vi "太阳能控制器MPPT24.vi"() -> ()   [LabVIEW 2016, in "环境动力监测库.lvlib"]
uses:
  <vilib>/Utility/miscctls.llb/LVPointTypeDef.ctl
  <vilib>/Utility/config.llb/NI_LVConfig.lvlib
  <vilib>/ptbypt/NI_PtbyPt.lvlib
panel:
  out "串口":string
  in  "串口启用 2":bool caption="串口启用"
  in  "报警设置":bool
  in  "MPPT-24 串口":refnum<visa-resource-name> caption="MPPT-24"
  out "充放电信息 2":T1 caption="充放电信息_KWH" {"总累计充电量" format="%.2f"; "当年累计充电量" format="%.2f"; "当月累计充电量" format="%.2f"; "当日累计充电量" format="%.2f"; "当年累计用电量" format="%.2f"; "当月累计用电量" format="%.2f"; "当日累计用电量" format="%.2f"}
  out "状态 2":string caption="状态"
  out "通讯状态 3":bool
  out "控制器信息 2":cluster{"设备温度℃":dbl} caption="控制器信息"
  out "直流负载信息 2":cluster{"负载电压V":dbl, "负载电流A":dbl, "负载功率W":dbl} caption="直流负载信息"
  out "蓄电池信息 2":T2 caption="蓄电池信息"
  out "阵列信息 2":cluster{"阵列电压V":dbl, "阵列电流A":dbl, "发电功率W":dbl} caption="阵列信息"
  # "MPPT-24"
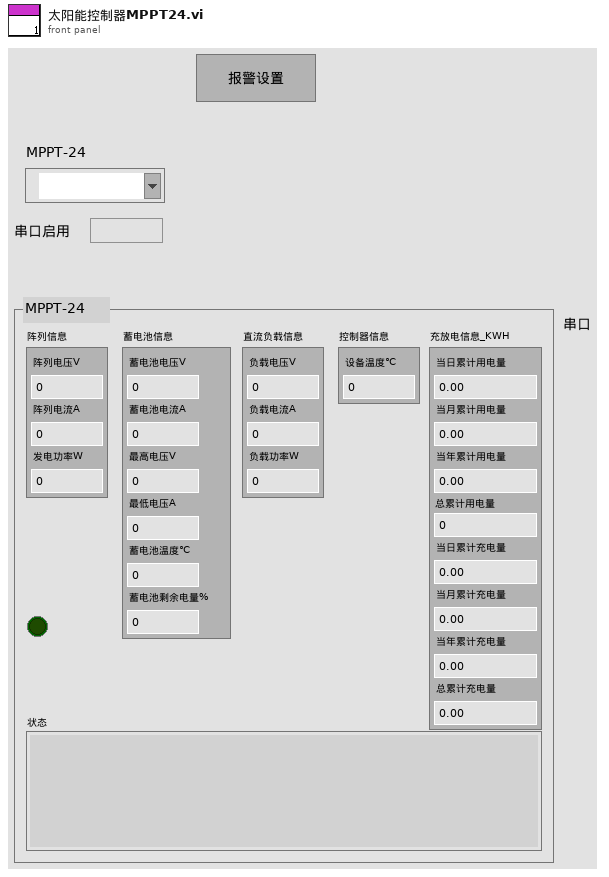
[diagram p1: front panel]
types:
  T1 = cluster{"当日累计用电量":sgl, "当月累计用电量":sgl, "当年累计用电量":sgl, "总累计用电量":sgl, "当日累计充电量":sgl, "当月累计充电量":sgl, "当年累计充电量":sgl, "总累计充电量":sgl}
  T2 = cluster{"蓄电池电压V":dbl, "蓄电池电流A":dbl, "最高电压V":dbl, "最低电压A":dbl, "蓄电池温度℃":dbl, "蓄电池剩余电量%":dbl}
  T3 = cluster{"baud rate (bps)":u32, "stop bits":u16, "parity":u16, "flow control":u16, "timeout":u32, "retries":i32}
  T4 = cluster{"监测项描述:输出":string, "连接方式":enum16{"串口", "TCP"}, "端口":string, "IP address:":string, "Port:":string, "站号":u64, "传感器型号":string, "波特率":u64, "data bits":u64, "停止位":u16, "奇偶校验":u16}
  T5 = typedef "LVPointTypeDef.ctl" = cluster{"Horizontal":i16, "Vertical":i16}
  T6 = cluster{"漏水监测输出":cluster{"漏水监测告警":bool, "告警内容":string}, "门禁监测输出":cluster{"门禁监测告警":bool, "告警内容":string}, "门禁监测输出2":cluster{"门禁监测告警":bool, "告警内容":string}, "温湿度监测输出":cluster{"温湿度监测告警":bool, "告警内容":string}, "烟雾监测输出":cluster{"烟雾监测告警":bool, "告警内容":string}, "空调监测输出":cluster{"空调监测告警":bool, "告警内容":string}, "自动重合闸输出":cluster{"自动重合闸告警":bool, "告警内容":string}, "红外入侵输出":cluster{"红外入侵告警":bool, "告警内容":string}, "振动输出":cluster{"振动告警":bool, "告警内容":string}, "UPS输出":cluster{"UPS告警":bool, "告警内容":string}, "蓄电池输出":cluster{"蓄电池告警":bool, "告警内容":string}, "蓄电池输出2":cluster{"蓄电池告警":bool, "告警内容":string}, "GPS输出":cluster{"定位告警":bool, "告警内容":string}, "北斗输出":cluster{"定位告警":bool, "告警内容":string}, "气象输出":cluster{"气象告警":bool, "告警内容":string}}
  T7 = cluster{"时间":timestamp, "阵列电压_V":dbl, "阵列电流_A":dbl, "发电功率_W":dbl, "蓄电池电压_V":dbl, "蓄电池电流_A":dbl, "最高电压_V":dbl, "最低电压_A":dbl, "蓄电池温度_℃":dbl, "蓄电池剩余电量_%":dbl, "负载电压_V":dbl, "负载电流_A":dbl, "负载功率_W":dbl, "设备温度_℃":dbl, "当日累计用电量_KWH":dbl, "当月累计用电量_KWH":dbl, "当年累计用电量_KWH":dbl, "总累计用电量_KWH":dbl, "当日累计充电量_KWH":dbl, "当月累计充电量_KWH":dbl, "当年累计充电量_KWH":dbl, "总累计充电量_KWH":dbl}
  T8 = typedef "LVDateTimeRec.ctl" = cluster{"秒数的小数部分":dbl, "秒":i32, "分":i32, "时":i32, "日":i32, "月":i32, "年":i32, "天数（周）":i32, "天数（年）":i32, "DST":i32}
  T9 = cluster{"市电":cluster{"状态":bool, "电压:":u16, "电流：":dbl, "详情  ":bool}, "UPS":cluster{"状态":bool, "输入电压:":sgl, "输出电压:":sgl, "电池电量:":u8, "电量":u16, "详情  ":bool}, "蓄电池12V":cluster{"状态":bool, "电压:":sgl, "电流:":sgl, "电池电量:":u8, "电量":u16, "详情  ":bool}, "蓄电池24V":cluster{"状态":bool, "电压:":sgl, "电流:":sgl, "电池电量:":u8, "电量":u16, "详情  ":bool}}
  T10 = cluster{"状态":cluster{"蓄电池状态":string, "阵列状态":string, "充电状态":string, "负载状态":string, "设备状态":string}, "充放电信息":cluster{"当日累计用电量":sgl, "当月累计用电量":sgl, "当年累计用电量":sgl, "总累计用电量":sgl, "当日累计充电量":sgl, "当月累计充电量":sgl, "当年累计充电量":sgl, "总累计充电量":sgl}, "控制器信息":cluster{"设备温度℃":dbl}, "蓄电池信息":cluster{"蓄电池电压V":dbl, "蓄电池电流A":dbl, "最高电压V":dbl, "最低电压A":dbl, "蓄电池温度℃":dbl, "蓄电池剩余电量%":dbl}, "阵列信息":cluster{"阵列电压V":dbl, "阵列电流A":dbl, "发电功率W":dbl}, "直流负载信息":cluster{"负载电压V":dbl, "负载电流A":dbl, "负载功率W":dbl}, "error out":errorcluster}
  T11 = enum32{"Bad", "Idle", "Run top level", "Running"}
  T12 = typedef "NI_LVConfig.lvlib/Config Data RefNum.ctl" = refnum<k1>
  T13 = enum8{"Enabled", "Disabled", "Disabled and Grayed Out"}
  T14 = cluster{"蓄电池状态":string, "阵列状态":string, "充电状态":string, "负载状态":string, "设备状态":string}
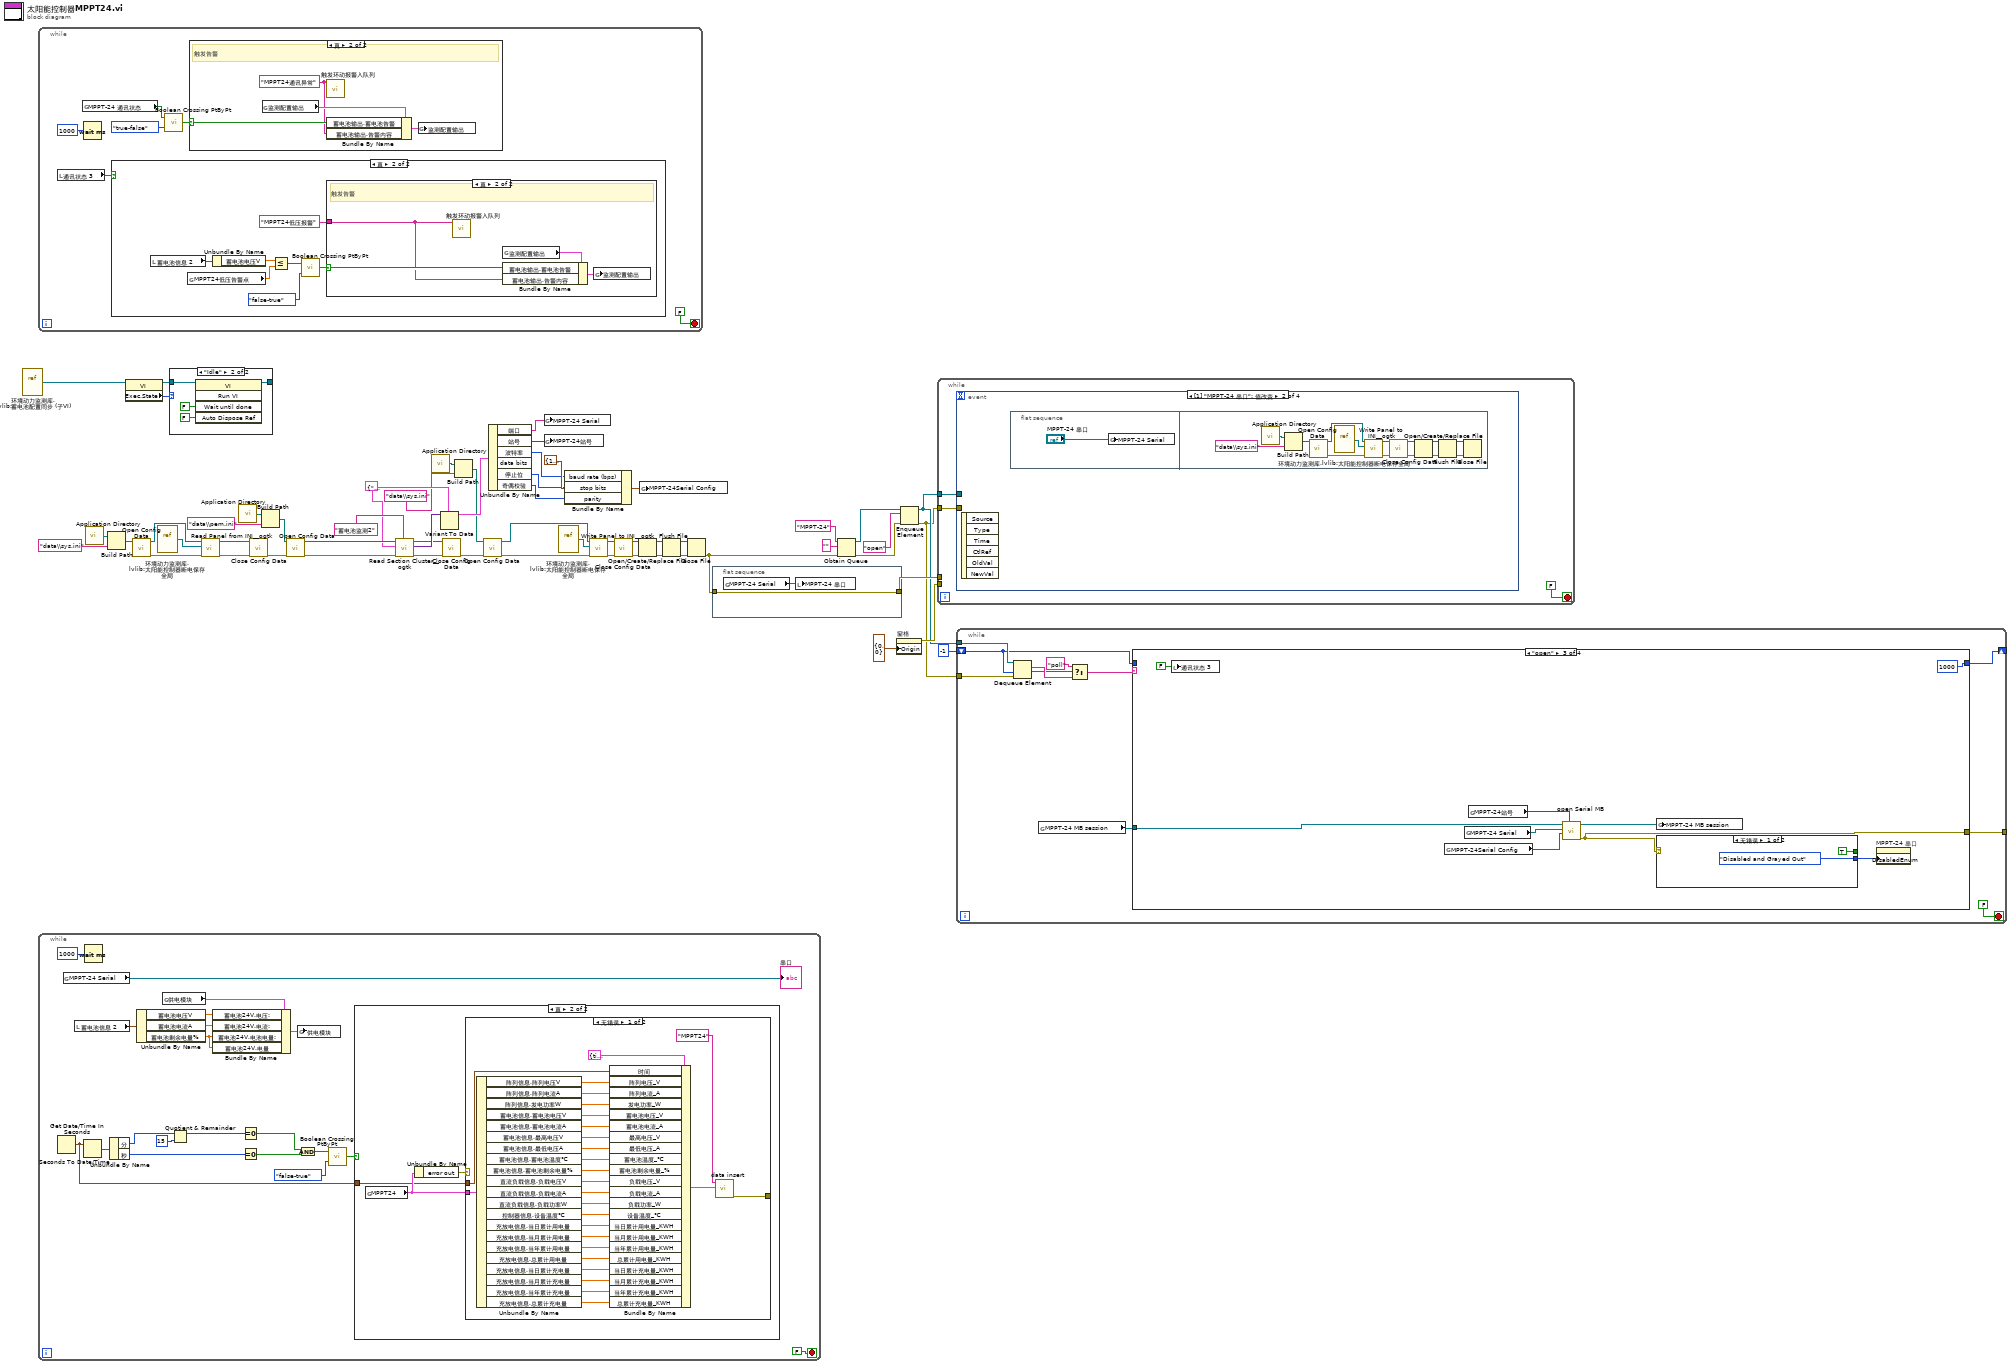
[diagram p0: block diagram]
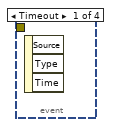
[diagram p8: hidden frame]
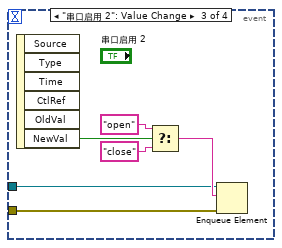
[diagram p9: hidden frame]
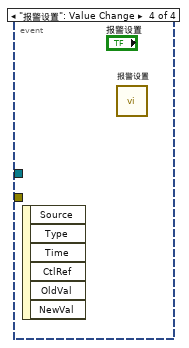
[diagram p10: hidden frame]
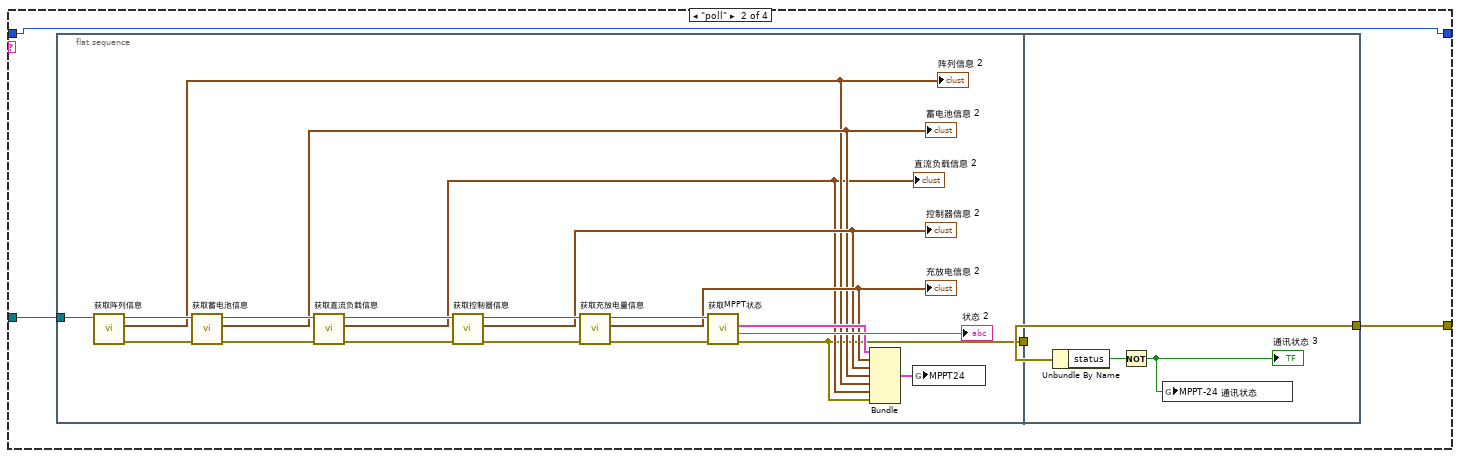
[diagram p12: hidden frame]
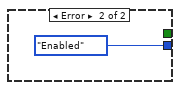
[diagram p13: hidden frame]
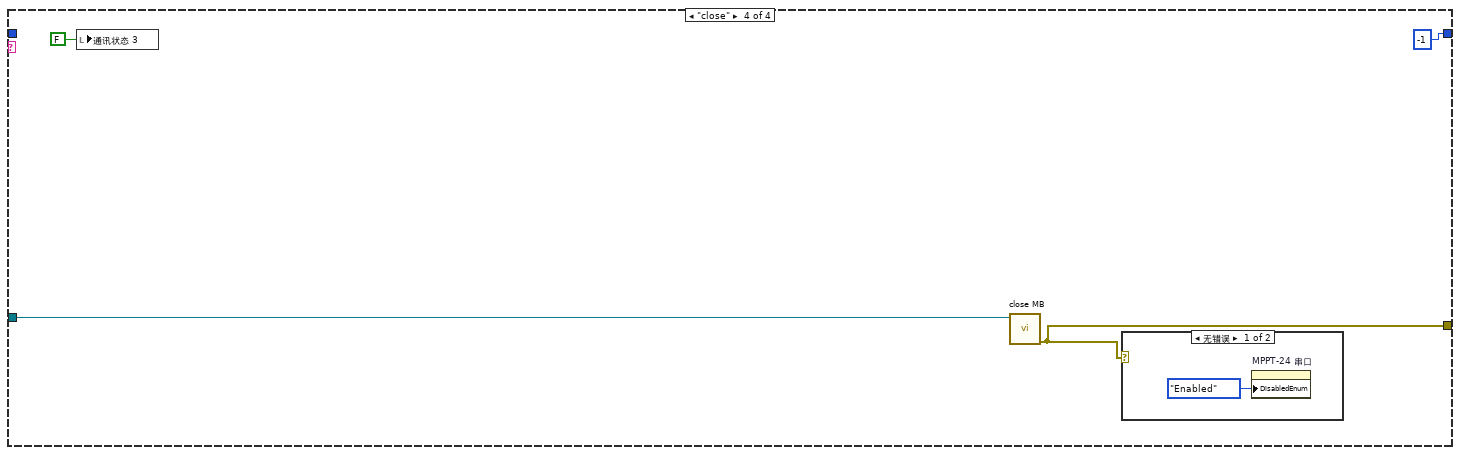
[diagram p14: hidden frame]
diagram:
  w36 = T4 {"监测项描述:输出"="", "连接方式"=enum."串口", "端口"="", "IP address:"="", "Port:"="", "站号"=19200, "传感器型号"="", "波特率"=19200, "data bits"=8, "停止位"=10, "奇偶校验"=0} ("输入簇")
  n1 = vi-ref "环境动力监测库.lvlib:蓄电池配置同步 (子VI).vi"() -> (w7:refnum<vi>)
  n2 = while {
    stop <- FALSE stop-if-true
    n3 = local read "通讯状态 3"() -> (w61:bool)
    n4 = global read "太阳能控制器全局.vi" "MPPT-24 通讯状态"() -> (w58:bool)
    n5 = Wait (ms)(milliseconds to wait=u32 1000 ("等待时间（毫秒）")) -> ()  [unwired: 1 out]
    n6 = case shown="真" w61 {
      frame False {
      }
      frame True {
        n7 = local read "蓄电池信息 2"() -> (w74:T2)
        n8 = global read "太阳能控制器断电保存全局.vi" "MPPT24低压告警点"() -> (w70:dbl)
        n9 = Unbundle By Name(w74) -> ("蓄电池电压V"=w71:dbl)
        n10 = Less Or Equal?(x=w71, y=w70) -> (x <= y?=w69:bool)
        n11 = call <vilib>:"Boolean Crossing PtByPt.vi"("direction"=enum16{"either", "false-true", "true-false"}."false-true", "input"=w69) -> ("crossing"=w72:bool)  [unwired: 1 in]
        n12 = case shown="真" w72 {
          selector: w72 -> [_ w76]
          tunnel: "MPPT24低压报警" ("设备") -> [_ w75]
          frame False {
          }
          frame True {
            # "触发告警"
            n13 = call "触发环动报警入队列.vi"("报警内容"=w75) -> ()  [unwired: 11 in]
            n14 = global read "断电保存全局变量.vi" "监测配置输出"() -> (w77:T6)
            n15 = Bundle By Name(cluster=w77, "蓄电池输出.蓄电池告警"=w76, "蓄电池输出.告警内容"=w75) -> (w78:T6)
            n16 = global write "断电保存全局变量.vi" "监测配置输出"(w78) -> ()
          }
        }
      }
    }
    n17 = call <vilib>:"Boolean Crossing PtByPt.vi"("direction"=enum16{"either", "false-true", "true-false"}."true-false", "input"=w58) -> ("crossing"=w59:bool)  [unwired: 1 in]
    n18 = case shown="真" w59 {
      selector: w59 -> [_ w65]
      frame False {
      }
      frame True {
        w64 = "MPPT24通讯异常" ("报警内容")
        # "触发告警"
        n19 = global read "断电保存全局变量.vi" "监测配置输出"() -> (w67:T6)
        n20 = call "触发环动报警入队列.vi"("报警内容"=w64) -> ()  [unwired: 11 in]
        n21 = Bundle By Name(cluster=w67, "蓄电池输出.蓄电池告警"=w65, "蓄电池输出.告警内容"=w64) -> (w66:T6)
        n22 = global write "断电保存全局变量.vi" "监测配置输出"(w66) -> ()
      }
    }
  }
  n23 = while {
    stop <- FALSE stop-if-true
    n24 = Get Date/Time In Seconds() -> (seconds since 1Jan1904=w86:timestamp)
    n25 = global read "太阳能控制器断电保存全局.vi" "MPPT-24 Serial"() -> (→"串口":refnum<visa-resource-name>)
    n26 = local read "蓄电池信息 2"() -> (w82:T2)
    n27 = Seconds To Date/Time(time stamp (now)=w86) -> (date time rec=w96:T8)  [unwired: 1 in]
    n28 = Wait (ms)(milliseconds to wait=u32 1000 ("等待时间（毫秒）")) -> ()  [unwired: 1 out]
    n29 = Unbundle By Name(w96) -> ("分"=w95:i32, "秒"=w92:i32)
    n30 = Unbundle By Name(w82) -> ("蓄电池电压V"=w81:dbl, "蓄电池电流A"=w80:dbl, "蓄电池剩余电量%"=w79:dbl)
    n31 = global read "内部交互全局变量.vi" "供电模块"() -> (w84:T9)
    n32 = Quotient & Remainder(x=w95, y=15) -> (x-y*floor(x/y)=w93:i32)  [unwired: 1 out]
    n33 = Bundle By Name(cluster=w84, "蓄电池24V.电压:"=w81, "蓄电池24V.电流:"=w80, "蓄电池24V.电池电量:"=w79, "蓄电池24V.电量"=w79) -> (w83:T9)
    n34 = Equal To 0?(x=w93) -> (x = 0?=w91:bool)
    n35 = Equal To 0?(x=w92) -> (x = 0?=w90:bool)
    n36 = global write "内部交互全局变量.vi" "供电模块"(w83) -> ()
    n37 = And(x=w91, y=w90) -> (x .and. y?=w89:bool)
    n38 = call <vilib>:"Boolean Crossing PtByPt.vi"("direction"=enum16{"either", "false-true", "true-false"}."false-true", "input"=w89) -> ("crossing"=w87:bool)  [unwired: 1 in]
    n39 = case shown="真" w87 {
      tunnel: w86 -> [_ w99]
      frame False {
      }
      frame True {
        n40 = global read "太阳能控制器全局.vi" "MPPT24"() -> (w101:T10)
        n41 = Unbundle By Name(w101) -> ("error out"=w100:errorcluster)
        n42 = case shown="无错误" w100 {
          tunnel: w101 -> [w106 _]
          tunnel: w99 -> [w105 _]
          tunnel: [w102 _] -> _
          frame No Error {
            n43 = Unbundle By Name(w106) -> ("阵列信息.阵列电压V"=w108:dbl, "阵列信息.阵列电流A"=w109:dbl, "阵列信息.发电功率W"=w110:dbl, "蓄电池信息.蓄电池电压V"=w111:dbl, "蓄电池信息.蓄电池电流A"=w112:dbl, "蓄电池信息.最高电压V"=w113:dbl, "蓄电池信息.最低电压A"=w114:dbl, "蓄电池信息.蓄电池温度℃"=w115:dbl, "蓄电池信息.蓄电池剩余电量%"=w116:dbl, "直流负载信息.负载电压V"=w117:dbl, "直流负载信息.负载电流A"=w118:dbl, "直流负载信息.负载功率W"=w119:dbl, "控制器信息.设备温度℃"=w120:dbl, "充放电信息.当日累计用电量"=w121:sgl, "充放电信息.当月累计用电量"=w122:sgl, "充放电信息.当年累计用电量"=w123:sgl, "充放电信息.总累计用电量"=w124:sgl, "充放电信息.当日累计充电量"=w125:sgl, "充放电信息.当月累计充电量"=w126:sgl, "充放电信息.当年累计充电量"=w127:sgl, "充放电信息.总累计充电量"=w128:sgl)
            n44 = Bundle By Name(cluster=T7 {"时间"=timestamp(0 s since 1904-01-01), "阵列电压_V"=0.0, "阵列电流_A"=0.0, "发电功率_W"=0.0, "蓄电池电压_V"=0.0, "蓄电池电流_A"=0.0, "最高电压_V"=0.0, "最低电压_A"=0.0, "蓄电池温度_℃"=0.0, "蓄电池剩余电量_%"=0.0, "负载电压_V"=0.0, "负载电流_A"=0.0, "负载功率_W"=0.0, "设备温度_℃"=0.0, "当日累计用电量_KWH"=0.0, "当月累计用电量_KWH"=0.0, "当年累计用电量_KWH"=0.0, "总累计用电量_KWH"=0.0, "当日累计充电量_KWH"=0.0, "当月累计充电量_KWH"=0.0, "当年累计充电量_KWH"=0.0, "总累计充电量_KWH"=0.0} ("data in"), "时间"=w105, "阵列电压_V"=w108, "阵列电流_A"=w109, "发电功率_W"=w110, "蓄电池电压_V"=w111, "蓄电池电流_A"=w112, "最高电压_V"=w113, "最低电压_A"=w114, "蓄电池温度_℃"=w115, "蓄电池剩余电量_%"=w116, "负载电压_V"=w117, "负载电流_A"=w118, "负载功率_W"=w119, "设备温度_℃"=w120, "当日累计用电量_KWH"=w121, "当月累计用电量_KWH"=w122, "当年累计用电量_KWH"=w123, "总累计用电量_KWH"=w124, "当日累计充电量_KWH"=w125, "当月累计充电量_KWH"=w126, "当年累计充电量_KWH"=w127, "总累计充电量_KWH"=w128) -> (w104:T7)
            n45 = call "data insert.vi"("data in"=w104, "table"="MPPT24") -> ("error out"=w102:errorcluster)  [unwired: 9 in]
          }
          frame Error {
          }
        }
      }
    }
  }
  n46 = call <vilib>:"Application Directory.vi"() -> ("Application Directory"=w13:path)
  n47 = Build Path(base path=w13, name or relative path="data\\sys.ini" ("名称或相对路径")) -> (appended path=w12:path)
  n48 = property class="VI"(reference=w7) -> (reference out=w8:refnum<vi>, "Exec.State"=w9:T11)  [unwired: 1 in, 1 out]
  n49 = call <vilib>:"Open Config Data.vi"("configuration file path"=w12) -> ("error out"=w16:errorcluster, "refnum"=w15:T12)  [unwired: 8 in, 1 out]
  n50 = vi-ref "环境动力监测库.lvlib:太阳能控制器断电保存全局.vi"() -> (w11:refnum<vi>)
  n51 = case shown="\"Idle\"" w9 {
    tunnel: w8 -> [w129 w131]
    tunnel: [w129 w130] -> _
    frame "Bad", Default {
    }
    frame "Idle" {
      n52 = invoke class="VI" method="Run VI"(reference=w131, "Wait until done"=FALSE ("结束前等待"), "Auto Dispose Ref"=FALSE ("自动销毁引用")) -> (reference out=w130:refnum<vi>)  [unwired: 2 in, 4 out]
    }
  }
  n53 = call <userlib>:"Read Panel from INI__ogtk.vi"("error in (no error)"=w16, "VI ref"=w11, "refnum"=w15) -> ("error out"=w18:errorcluster, "refnum out"=w17:T12)  [unwired: 7 in]
  n54 = call <vilib>:"Application Directory.vi"() -> ("Application Directory"=w40:path)
  n55 = call <vilib>:"Close Config Data.vi"("error in (no error)"=w18, "refnum"=w17) -> ("error out"=w10:errorcluster)  [unwired: 8 in, 1 out]
  n56 = Build Path(base path=w40, name or relative path="data\\pem.ini" ("名称或相对路径")) -> (appended path=w39:path)
  n57 = call <vilib>:"Open Config Data.vi"("error in (no error)"=w10, "configuration file path"=w39) -> ("error out"=w38:errorcluster, "refnum"=w37:T12)  [unwired: 7 in, 1 out]
  n58 = call <userlib>:"Read Section Cluster__ogtk.vi"("section (optional)"="蓄电池监测2", "error in (no error)"=w38, "Section Formatted Cluster Type"=w36, "refnum"=w37) -> ("error out"=w44:errorcluster, "Section Formatted Cluster"=w45:variant, "dup refnum"=w43:T12)  [unwired: 3 in, 2 out]
  n59 = call <vilib>:"Application Directory.vi"() -> ("Application Directory"=w34:path)
  n60 = Variant To Data(type=w36, Variant=w45) -> (data=w46:T4)  [unwired: 1 in, 1 out]
  n61 = call <vilib>:"Close Config Data.vi"("error in (no error)"=w44, "refnum"=w43) -> ("error out"=w22:errorcluster)  [unwired: 8 in, 1 out]
  n62 = Build Path(base path=w34, name or relative path="data\\sys.ini" ("名称或相对路径")) -> (appended path=w33:path)
  n63 = call <vilib>:"Open Config Data.vi"("error in (no error)"=w22, "configuration file path"=w33) -> ("error out"=w30:errorcluster, "refnum"=w32:T12)  [unwired: 7 in, 1 out]
  n64 = Unbundle By Name(w46) -> ("端口"=w20:string, "站号"=w5:u64, "波特率"=w4:u64, "停止位"=w3:u16, "奇偶校验"=w2:u16)  [unwired: 1 out]
  n65 = global write "太阳能控制器断电保存全局.vi" "MPPT-24 Serial"(w20) -> ()
  n66 = global write "太阳能控制器断电保存全局.vi" "MPPT-24站号"(w5) -> ()
  n67 = vi-ref "环境动力监测库.lvlib:太阳能控制器断电保存全局.vi"() -> (w21:refnum<vi>)
  n68 = Bundle By Name(cluster=T3 {"baud rate (bps)"=115200, "stop bits"=10, "parity"=0, "flow control"=0, "timeout"=1000, "retries"=1} ("MPPT-24Serial Config"), "baud rate (bps)"=w4, "stop bits"=w3, "parity"=w2) -> (w1:T3)
  n69 = call <userlib>:"Write Panel to INI__ogtk.vi"("error in (no error)"=w30, "VI ref"=w21, "refnum"=w32) -> ("error out"=w29:errorcluster, "refnum out"=w31:T12)  [unwired: 7 in]
  n70 = call <vilib>:"Close Config Data.vi"("error in (no error)"=w29, "refnum"=w31) -> ("error out"=w24:errorcluster, "file path"=w23:path)  [unwired: 8 in]
  n71 = Open/Create/Replace File(file path (use dialog)=w23, error in=w24) -> (refnum out=w27:refnum<file>, error out=w28:errorcluster)  [unwired: 4 in, 1 out]
  n72 = global write "太阳能控制器断电保存全局.vi" "MPPT-24Serial Config"(w1) -> ()
  n73 = Flush File(refnum=w27, error in=w28) -> (refnum out=w26:refnum<file>, error out=w25:errorcluster)
  n74 = Close File(refnum=w26, error in=w25) -> (error out=w19:errorcluster)  [unwired: 1 out]
  n75 = flat-sequence {
    tunnel: w19 -> [w134]
    tunnel: [w134] -> w49
    frame #0 {
      n76 = global read "太阳能控制器断电保存全局.vi" "MPPT-24 Serial"() -> (w135:refnum<visa-resource-name>)
      n77 = local write "MPPT-24 串口"(w135) -> ()
    }
  }
  n78 = Obtain Queue(name (unnamed)="MPPT-24" ("名称（未命名）"), element data type="", error in (no error)=w19) -> (queue out=w51:refnum<queue>, error out=w50:errorcluster)  [unwired: 2 in, 1 out]
  n79 = property on="窗格" class="Pane"("Origin"=T5 {"Horizontal"=0, "Vertical"=0} ("原点")) -> (error out=w55:errorcluster)  [unwired: 2 in, 1 out]
  n80 = Enqueue Element(queue=w51, element="open" ("元素"), error in (no error)=w50) -> (queue out=w48:refnum<queue>, error out=w47:errorcluster)  [unwired: 1 in, 1 out]
  n81 = while {
    tunnel: w55 -> [_]
    tunnel: w49 -> [_]
    tunnel: w48 -> [w137]
    tunnel: w47 -> [w136]
    stop <- FALSE stop-if-true
    n82 = event shown="[1] \"MPPT-24 串口\": 值改变" {
      selector: _ -> [_ _ _ _]
      dyn-events: _ -> [_ _ _ _]
      timeout: _ -> [_ _ _ _]
      tunnel: w137 -> [_ _ w155 _]
      tunnel: w136 -> [_ _ w154 _]
      event Timeout {
        n83 = event-data() -> ()  [unwired: 1 in, 3 out]
      }
      event "MPPT-24 串口": Value Change {
        n84 = event-data() -> ()  [unwired: 1 in, 6 out]
        n85 = flat-sequence {
          frame #0 {
            n86 = global write "太阳能控制器断电保存全局.vi" "MPPT-24 Serial"("MPPT-24 串口") -> ()
          }
          frame #1 {
            n87 = call <vilib>:"Application Directory.vi"() -> ("Application Directory"=w153:path)
            n88 = Build Path(base path=w153, name or relative path="data\\sys.ini" ("名称或相对路径")) -> (appended path=w151:path)
            n89 = call <vilib>:"Open Config Data.vi"("configuration file path"=w151) -> ("error out"=w147:errorcluster, "refnum"=w150:T12)  [unwired: 8 in, 1 out]
            n90 = vi-ref "环境动力监测库.lvlib:太阳能控制器断电保存全局.vi"() -> (w149:refnum<vi>)
            n91 = call <userlib>:"Write Panel to INI__ogtk.vi"("error in (no error)"=w147, "VI ref"=w149, "refnum"=w150) -> ("error out"=w146:errorcluster, "refnum out"=w148:T12)  [unwired: 7 in]
            n92 = call <vilib>:"Close Config Data.vi"("error in (no error)"=w146, "refnum"=w148) -> ("error out"=w141:errorcluster, "file path"=w140:path)  [unwired: 8 in]
            n93 = Open/Create/Replace File(file path (use dialog)=w140, error in=w141) -> (refnum out=w144:refnum<file>, error out=w145:errorcluster)  [unwired: 4 in, 1 out]
            n94 = Flush File(refnum=w144, error in=w145) -> (refnum out=w143:refnum<file>, error out=w142:errorcluster)
            n95 = Close File(refnum=w143, error in=w142) -> ()  [unwired: 2 out]
          }
        }
      }
      event "串口启用 2": Value Change {
        n96 = event-data() -> ("NewVal"=w156:bool)  [unwired: 1 in, 5 out]
        n97 = Select(t="open", s=w156, f="close") -> (s? t:f=w158:string)
        n98 = Enqueue Element(queue=w155, element=w158, error in (no error)=w154) -> ()  [unwired: 1 in, 3 out]
      }
      event "报警设置": Value Change {
        n99 = event-data() -> ()  [unwired: 1 in, 6 out]
        n100 = call "报警设置.vi"() -> ()  [unwired: 12 in]
      }
    }
  }
  n101 = while {
    tunnel: w48 -> [w167]
    tunnel: w47 -> [w166]
    shift-right: [w162] -> _
    shift-left: -1 ("超时毫秒(-1)") -> [w160]
    tunnel: [w163] -> _
    stop <- FALSE stop-if-true
    n102 = Dequeue Element(queue=w167, timeout in ms (-1)=w160, error in (no error)=w166) -> (element=w170:string, timed out?=w168:bool)  [unwired: 2 out]
    n103 = global read "太阳能控制器全局.vi" "MPPT-24 MB session"() -> (w164:refnum<class "MB_Master.lvclass">)
    n104 = Select(t="poll" ("元素"), s=w168, f=w170) -> (s? t:f=w165:string)
    n105 = case shown="\"open\"" w165 {
      tunnel: w164 -> [_ w175 w204 w213]
      tunnel: [_ w173 w203 w212] -> w163
      tunnel: [w171 w172 1000 ("超时毫秒(-1)") -1 ("超时毫秒(-1)")] -> w162
      tunnel: w160 -> [w171 w172 _ _]
      frame Default {
      }
      frame "poll" {
        n106 = flat-sequence {
          tunnel: w175 -> [w185]
          tunnel: [w176] -> w174
          tunnel: w174 -> [w196]
          tunnel: [w196] -> w173
          frame #0 {
            n107 = call "获取阵列信息.vi"("MB session in"=w185) -> ("error out"=w194:errorcluster, "阵列信息"=w178:cluster{"阵列电压V":dbl, "阵列电流A":dbl, "发电功率W":dbl}, "MB session out"=w195:refnum<class "MB_Master.lvclass">)  [unwired: 8 in]
            "阵列信息 2" <- w178
            n108 = call "获取蓄电池信息.vi"("error in (no error)"=w194, "MB session in"=w195) -> ("error out"=w192:errorcluster, "蓄电池信息"=w179:T2, "MB session out"=w193:refnum<class "MB_Master.lvclass">)  [unwired: 7 in]
            "蓄电池信息 2" <- w179
            n109 = call "获取直流负载信息.vi"("error in (no error)"=w192, "MB session in"=w193) -> ("error out"=w190:errorcluster, "直流负载信息"=w177:cluster{"负载电压V":dbl, "负载电流A":dbl, "负载功率W":dbl}, "MB session out"=w191:refnum<class "MB_Master.lvclass">)  [unwired: 7 in]
            "直流负载信息 2" <- w177
            n110 = call "获取控制器信息.vi"("error in (no error)"=w190, "MB session in"=w191) -> ("error out"=w188:errorcluster, "控制器信息"=w180:cluster{"设备温度℃":dbl}, "MB session out"=w189:refnum<class "MB_Master.lvclass">)  [unwired: 7 in]
            "控制器信息 2" <- w180
            n111 = call "获取充放电量信息.vi"("error in (no error)"=w188, "MB session in"=w189) -> ("error out"=w186:errorcluster, "充放电信息"=w181:T1, "MB session out"=w187:refnum<class "MB_Master.lvclass">)  [unwired: 7 in]
            "充放电信息 2" <- w181
            n112 = call "获取MPPT状态.vi"("error in (no error)"=w186, "MB session in"=w187) -> ("error out"=w176:errorcluster, "结果字符串"=→"状态 2":string, "状态"=w183:T14)  [unwired: 6 in, 1 out]
            n113 = Bundle("状态"=w183, "充放电信息"=w181, "控制器信息"=w180, "蓄电池信息"=w179, "阵列信息"=w178, "直流负载信息"=w177, "error out"=w176) -> (w182:T10)  [unwired: 1 in]
            n114 = global write "太阳能控制器全局.vi" "MPPT24"(w182) -> ()
          }
          frame #1 {
            n115 = Unbundle By Name(w196) -> ("status"=w198:bool)
            n116 = Not(x=w198) -> (.not. x?=w197:bool)
            "通讯状态 3" <- w197
            n117 = global write "太阳能控制器全局.vi" "MPPT-24 通讯状态"(w197) -> ()
          }
        }
      }
      frame "open" {
        n118 = local write "通讯状态 3"(FALSE ("通讯状态 3")) -> ()
        n119 = global read "太阳能控制器断电保存全局.vi" "MPPT-24Serial Config"() -> (w200:T3)
        n120 = global read "太阳能控制器断电保存全局.vi" "MPPT-24 Serial"() -> (w205:refnum<visa-resource-name>)
        n121 = global read "太阳能控制器断电保存全局.vi" "MPPT-24站号"() -> (w199:u64)
        n122 = call "open Serial MB.vi"("Slave ID"=w199, "Serial Config"=w200, "VISA Resource"=w205, "MB session in"=w204) -> ("error out"=w203:errorcluster, "MB session out"=w206:refnum<class "MB_Master.lvclass">)  [unwired: 6 in]
        n123 = global write "太阳能控制器全局.vi" "MPPT-24 MB session"(w206) -> ()
        n124 = case shown="无错误" w203 {
          tunnel: [T13."Disabled and Grayed Out" ("禁用") T13."Enabled" ("禁用")] -> w201
          tunnel: [TRUE _] -> _
          frame No Error {
          }
          frame Error {
          }
        }
        n125 = property on="MPPT-24 串口" class="VISAName"("DisabledEnum"=w201) -> ()  [unwired: 2 in, 2 out]
      }
      frame "close" {
        n126 = local write "通讯状态 3"(FALSE ("通讯状态 2")) -> ()
        n127 = call "close MB.vi"("MB session in"=w213) -> ("error out"=w212:errorcluster)  [unwired: 10 in]
        n128 = case shown="无错误" w212 {
          frame No Error {
            n129 = property on="MPPT-24 串口" class="VISAName"("DisabledEnum"=T13."Enabled" ("禁用")) -> ()  [unwired: 2 in, 2 out]
          }
          frame Error {
          }
        }
      }
    }
  }
